vi "Test-client-limit.vi"(8 "error in (no error)":errorcluster, 10 "Module type":T1=enum."Server", 11 "ModComm in":T2) -> (0 "error out":errorcluster, 1 "Client allowed?":bool, 2 "Module type dup":T1=enum."Server", 3 "ModComm out":T2)   [LabVIEW 2013, in "SLMServer.lvlib" / "SLMServer.lvclass"]
uses:
  SLMServer.lvclass
  Object-reference.ctl
  Supported-module-types.ctl
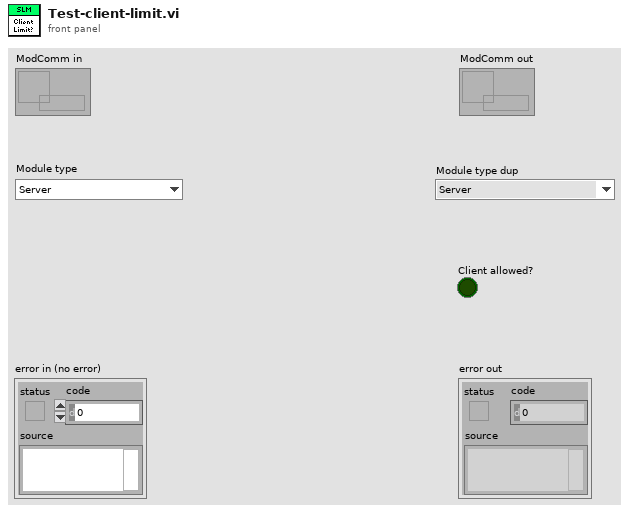
[diagram p1: front panel]
types:
  T1 = typedef "SLMServer.lvlib/SLMServer.lvclass/Supported-module-types.ctl" = enum16{"SLMControl", "PowderDeposition", "CameraVision", "Server", "All", "StrategyParser", "MaterialCharacterization", "StatusMonitor", "SLMSimulation", "LaserCharacterization"}
  T2 = typedef "SLMServer.lvlib/SLMServer.lvclass/Object-reference.ctl" = refnum<data-value>
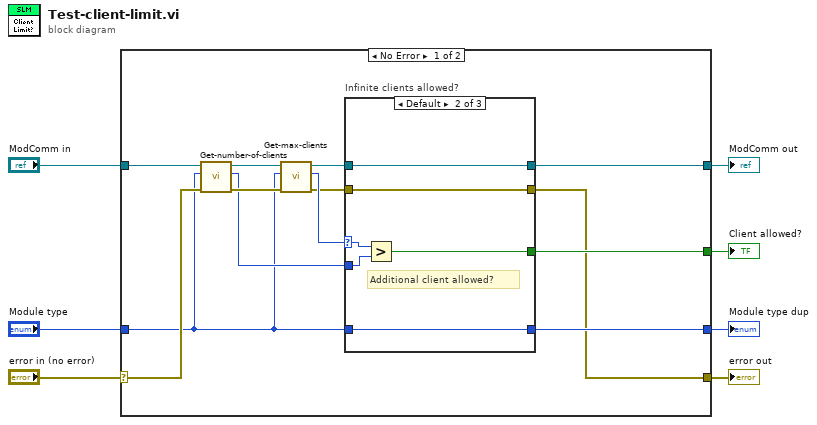
[diagram p0: block diagram]
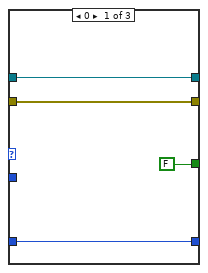
[diagram p2: hidden frame]
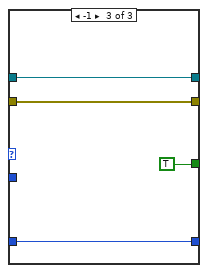
[diagram p3: hidden frame]
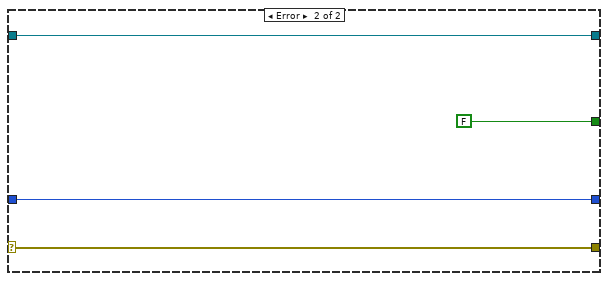
[diagram p4: hidden frame]
diagram:
  n1 = case shown="No Error" "error in (no error)" {
    selector: "error in (no error)" -> [w15 w38]
    tunnel: [w8 w38] -> w6
    tunnel: [w9 w37] -> w4
    tunnel: "ModComm in" -> [w20 w37]
    tunnel: "Module type" -> [w12 w35]
    tunnel: [w11 FALSE] -> w2
    tunnel: [w10 w35] -> w1
    frame No Error {
      n2 = call "Get-number-of-clients.vi"("error in (no error)"=w15, "Module type"=w12, "ModComm in"=w20) -> ("error out"=w18:errorcluster, "# clients"=w16:i32, "ModComm out"=w19:T2)  [unwired: 6 in]
      n3 = call "Get-max-clients.vi"("error in (no error)"=w18, "Module type"=w12, "ModComm in"=w19) -> ("error out"=w13:errorcluster, "Max clients"=w17:i32, "ModComm out"=w14:T2)  [unwired: 6 in]
      n4 = case "Infinite clients allowed?" shown="Default" w17 {
        selector: w17 -> [_ w30 _]
        tunnel: w16 -> [_ w29 _]
        tunnel: [FALSE w28 TRUE] -> w11
        tunnel: w14 -> [w22 w27 w33]
        tunnel: w13 -> [w21 w26 w32]
        tunnel: w12 -> [w23 w25 w31]
        tunnel: [w22 w27 w33] -> w9
        tunnel: [w21 w26 w32] -> w8
        tunnel: [w23 w25 w31] -> w10
        frame 0 {
        }
        frame Default {
          # "Additional client allowed?"
          n5 = Greater?(x=w30, y=w29) -> (0:w28:bool)
        }
        frame -1 {
        }
      }
    }
    frame Error {
    }
  }
  "error out" <- w6
  "ModComm out" <- w4
  "Client allowed?" <- w2
  "Module type dup" <- w1
